vi "Force_reference_L.vi"(1 "Force_peak":sgl, 11 "에러 출력":errorcluster) -> (4 "Force_Reference_L":sgl, 8 "출력 클러스터 3":T1, 15 "에러 출력 2":errorcluster caption="에러 입력(에러 없음)")   [LabVIEW 2019]
uses:
  1716bd58-37a0-4d94-8de8-90046bc3344a.vi
  <vilib>/Analysis/NI_AALBase.lvlib
  <vilib>/Analysis/baseanly.llb/Mean (DBL).vi
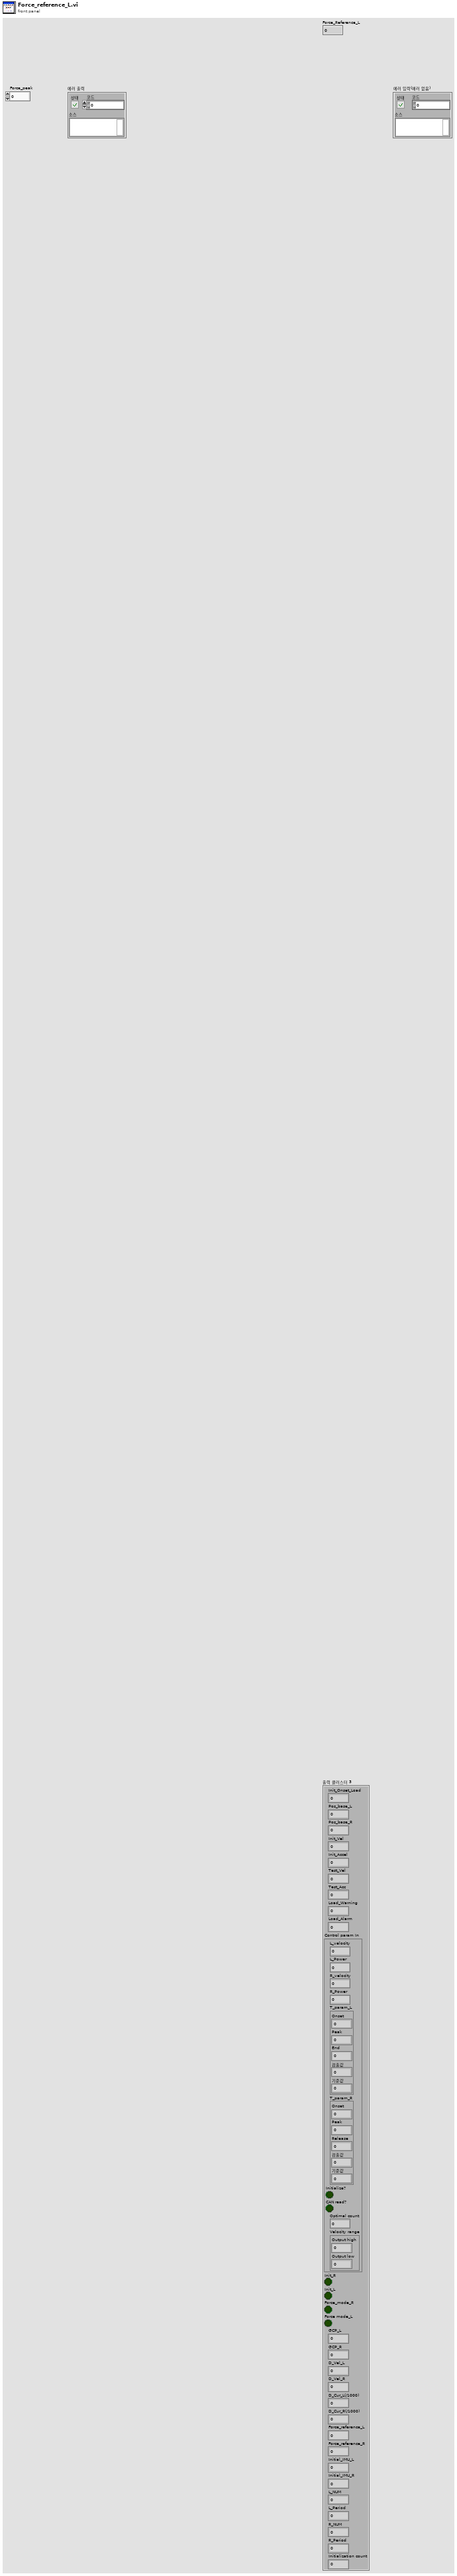
[diagram p1: front panel]
types:
  T1 = cluster{"Init_Onset_Load":sgl, "Pos_base_L":sgl, "Pos_base_R":sgl, "Init_Vel":i32, "Init_Accel":u32, "Test_Vel":i32, "Test_Acc":u32, "Load_Warning":sgl, "Load_Alarm":sgl, "Control param In":cluster{"L_velocity":u32, "L_Power":sgl, "R_velocity":u32, "R_Power":sgl, "T_param_L":cluster{"Onset":sgl, "Peak":sgl, "End":sgl, "검출값":sgl, "기준값":sgl}, "T_param_R":cluster{"Onset":sgl, "Peak":sgl, "Release":sgl, "검출값":sgl, "기준값":sgl}, "Initialize?":bool, "CAN read?":bool, "Optimal count":i32, "Velocity range":cluster{"Output high":dbl, "Output low":dbl}}, "Init_R":bool, "Init_L":bool, "Force_mode_R":bool, "Force mode_L":bool, "GCP_L":sgl, "GCP_R":sgl, "D_Vel_L":sgl, "D_Vel_R":sgl, "D_Cur_L(/1000)":sgl, "D_Cur_R(/1000)":sgl, "Force_reference_L":sgl, "Force_reference_R":sgl, "Initial_IMU_L":sgl, "Initial_IMU_R":sgl, "L_NUM":u32, "L_Period":i16, "R_NUM":u32, "R_Period":i16, "Initialization count":i32}
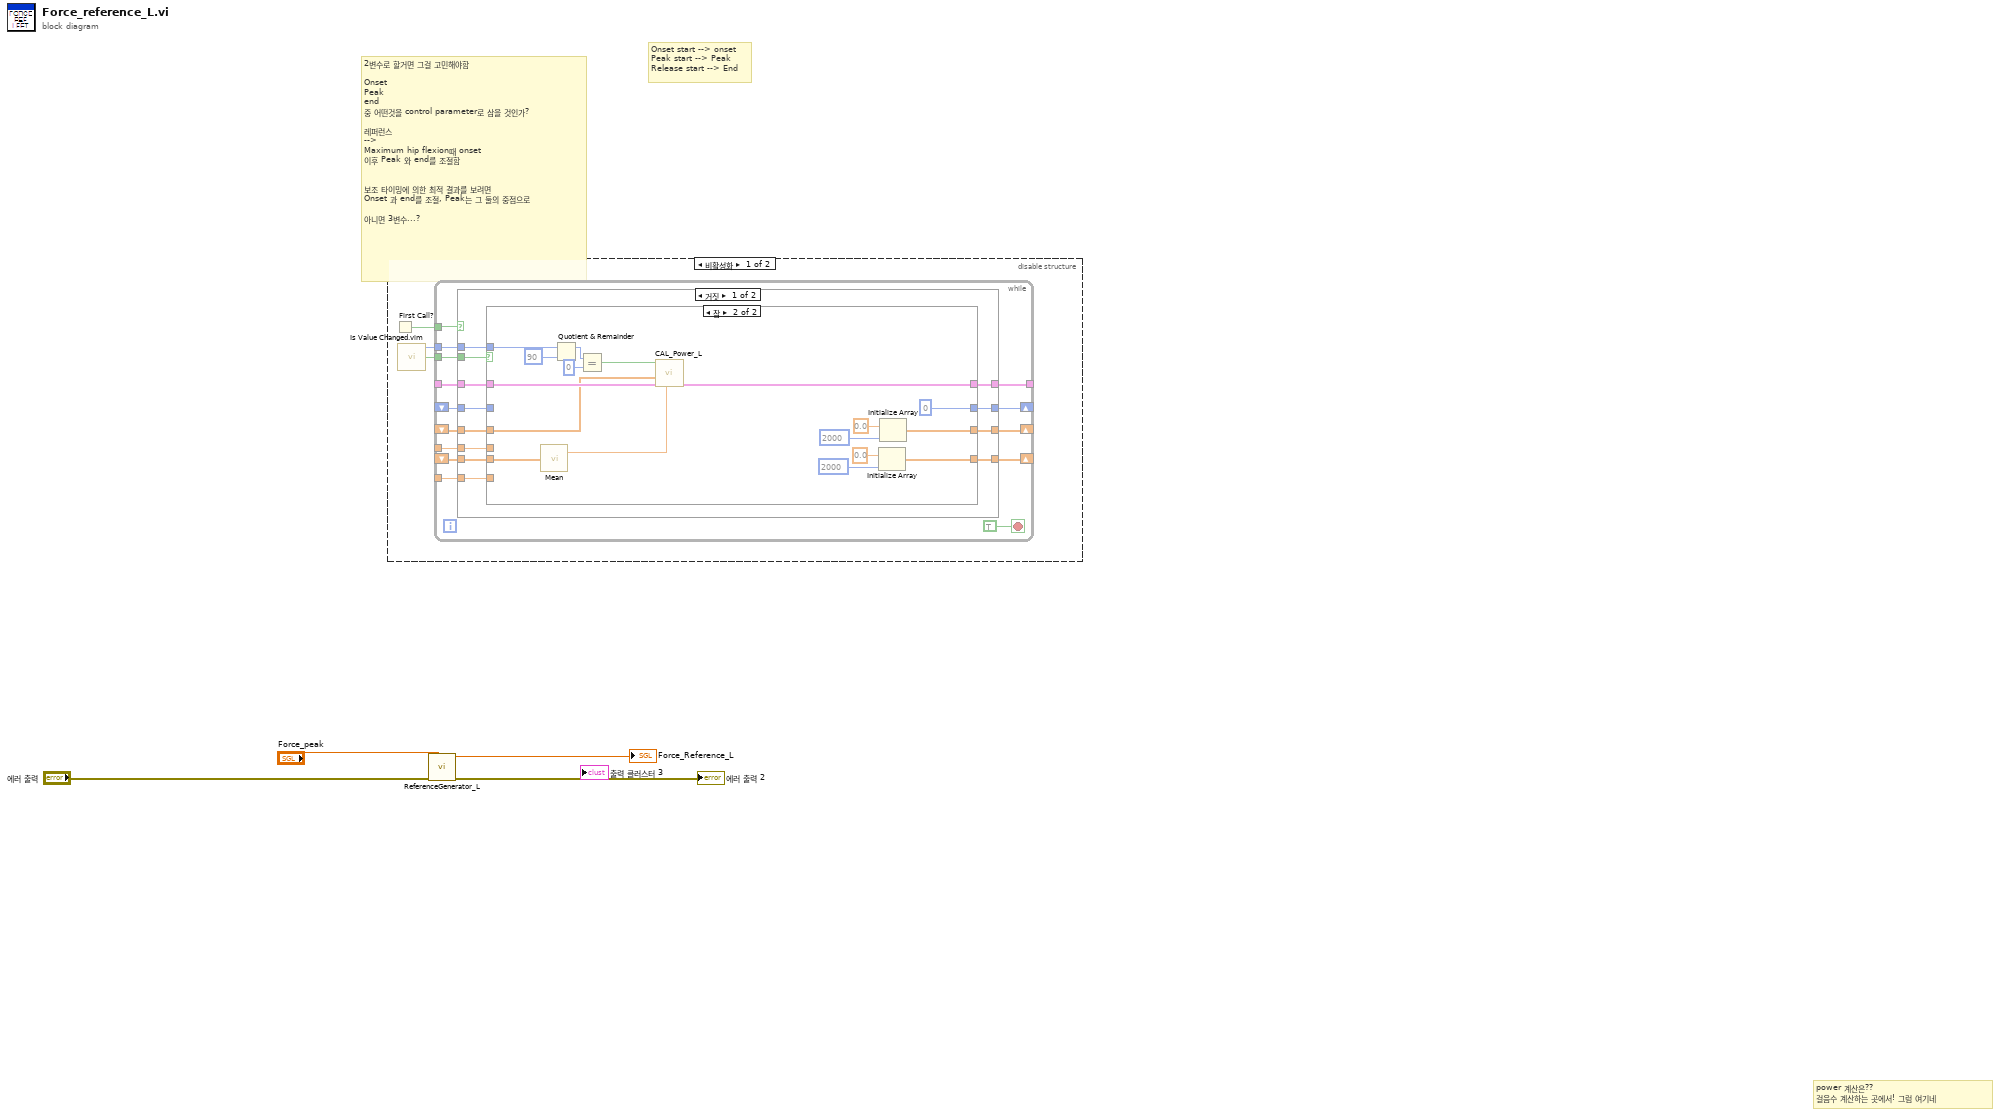
[diagram p0: block diagram]
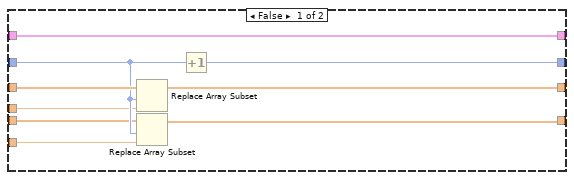
[diagram p2: hidden frame]
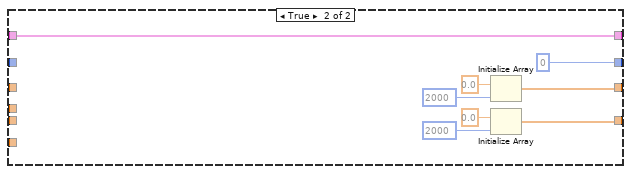
[diagram p3: hidden frame]
diagram:
  # "power 계산은??\n걸음수 계산하는 곳에서! 그럼 여기네"
  # "Onset start --> onset\nPeak start --> Peak\nRelease start --> End"
  # "2변수로 할거면 그걸 고민해야함\n\nOnset\nPeak \nend \n중 어떤것을 control parameter로 삼을 것인가?\n\n레퍼런스\n--> \nMaximum hip flexion때 onset\n이후 Peak 와 end를 조절함\n\n\n보조 타이밍에 의한 최적 결과를 보려면\nOnset 과 end를 조절, Peak는 그 둘의 중점으로\n\n아니면 3변수...?"
  n1 = disable-structure shown="비활성화" {
    frame Disabled {
      n2 = First Call?() -> (First Call?: T/F=w7:bool)
      n3 = call "Is Value Changed.vim"() -> ("changed or first call?"=w6:bool, "value"=w5:u32)
      n4 = while {
        tunnel: w7 -> [w20]
        tunnel: w6 -> [w19]
        shift-right: [w18] -> _
        shift-left: _ -> [w15]
        shift-right: [w17] -> _
        shift-left: _ -> [w14]
        shift-right: [w16] -> _
        shift-left: _ -> [w13]
        tunnel: _ -> [w12]
        tunnel: _ -> [w11]
        tunnel: _ -> [w10]
        tunnel: w5 -> [w9]
        tunnel: [w8] -> _
        stop <- TRUE stop-if-true
        n5 = case shown="거짓" w20 {
          tunnel: w19 -> [w33 _]
          tunnel: [w32 w65] -> w18
          tunnel: [w31 0] -> w17
          tunnel: [w30 w61] -> w16
          tunnel: w15 -> [w29 _]
          tunnel: w14 -> [w28 _]
          tunnel: w13 -> [w27 _]
          tunnel: w12 -> [w26 _]
          tunnel: w11 -> [w25 _]
          tunnel: w10 -> [w24 w60]
          tunnel: w9 -> [w23 _]
          tunnel: [w22 w60] -> w8
          frame False {
            n6 = case shown="참" w33 {
              tunnel: [w40 w57] -> w32
              tunnel: [w41 0] -> w31
              tunnel: [w37 w53] -> w30
              tunnel: w29 -> [w42 w44]
              tunnel: w28 -> [w39 _]
              tunnel: w27 -> [w38 w52]
              tunnel: w26 -> [w36 _]
              tunnel: w25 -> [w35 _]
              tunnel: w24 -> [w34 w50]
              tunnel: w23 -> [_ w46]
              tunnel: [w34 w43] -> w22
              frame False {
                n7 = Replace Array Subset(array=w42, new element=w36, index=w39) -> (w40:sgl[])
                n8 = Replace Array Subset(array=w38, new element=w35, index=w39) -> (w37:sgl[])
                n9 = Increment(x=w39) -> (x+1=w41:i32)
              }
              frame True {
                n10 = call-poly <vilib>:"Mean.vi"("X"=w52) -> ("mean"=w51:dbl)  [unwired: 1 out]
                n11 = Quotient & Remainder(x=w46, y=u32 90) -> (x-y*floor(x/y)=w49:u32)  [unwired: 1 out]
                n12 = Equal?(x=w49, y=u32 0) -> (x = y?=w45:bool)
                n13 = call "CAL_Power_L.vi"("stride?"=w45, "Positive Power"=w44, "출력 클러스터 2"=w50, "Period_L"=w51) -> ("출력 클러스터 3"=w43:T1)  [unwired: 6 in]
                n14 = Initialize Array(sgl 0.0 ("원소"), 2000 ("차원 크기")) -> (w53:sgl[])
                n15 = Initialize Array(sgl 0.0 ("원소"), 2000 ("차원 크기")) -> (w57:sgl[])
              }
            }
          }
          frame True {
            n16 = Initialize Array(sgl 0.0 ("원소"), 2000 ("차원 크기")) -> (w65:sgl[])
            n17 = Initialize Array(sgl 0.0 ("원소"), 2000 ("차원 크기")) -> (w61:sgl[])
          }
        }
      }
    }
    frame Enabled {
    }
  }
  n18 = call "ReferenceGenerator_L.vi"(1:"Force_peak", "에러 출력"="에러 출력") -> ("Force_Reference_L"=→"Force_Reference_L":sgl, "에러 출력 2"=→"에러 출력 2":errorcluster)  [unwired: 11 in, 1 out]
